vi "Step2.vi"(7 "Count In":i64, 8 "End":cluster{"Row":i32, "Col":i32}, 10 "Grid":string[][](array[string]), 11 "Current Pos":cluster{"Row":i32, "Col":i32}) -> (3 "Counts Out":i64[](array[numeric]))   [LabVIEW 2021]
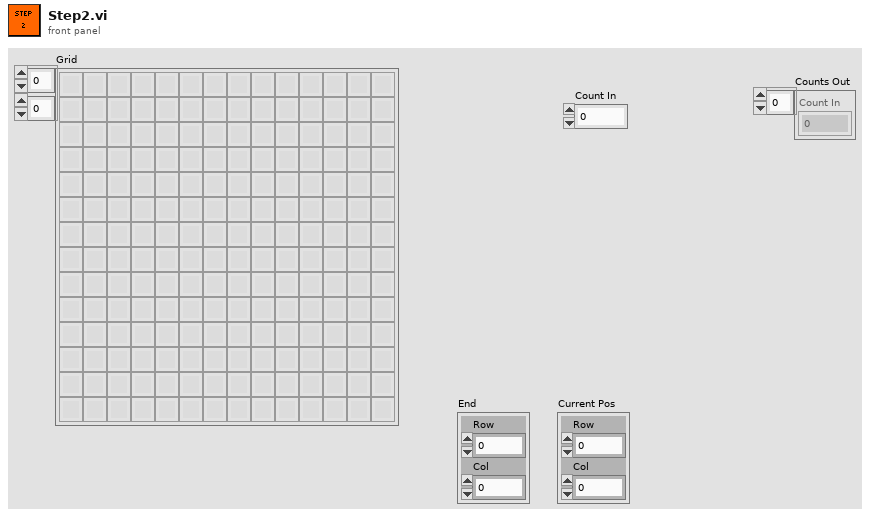
[diagram p1: front panel]
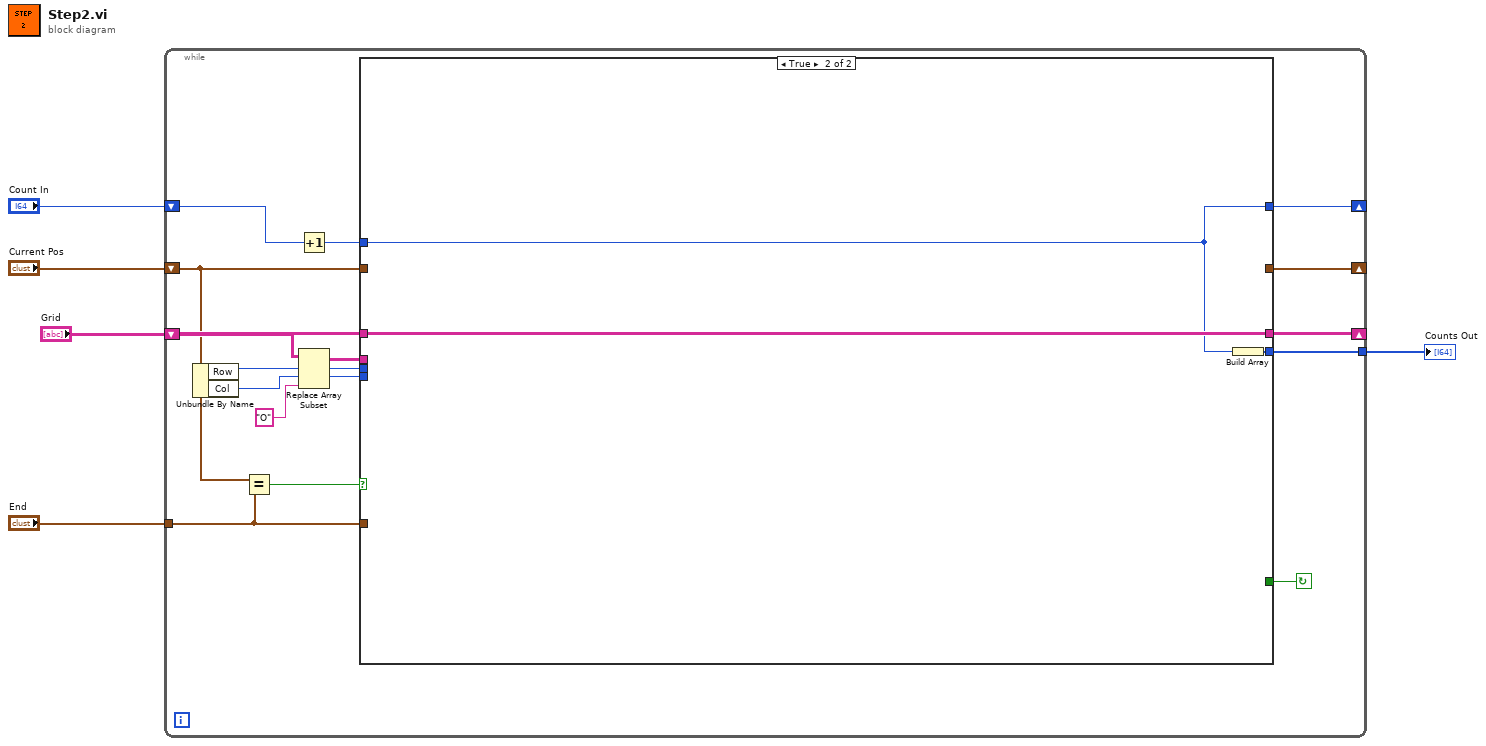
[diagram p0: block diagram]
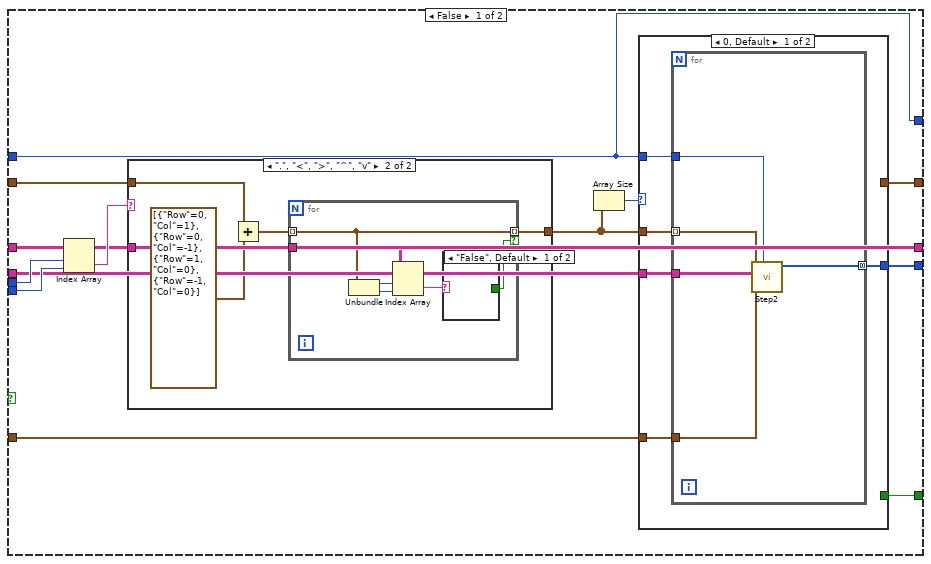
[diagram p2: hidden frame]
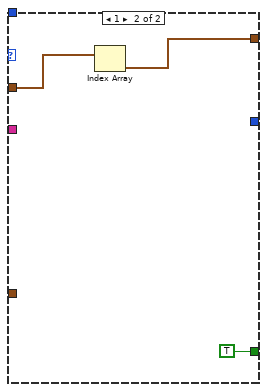
[diagram p3: hidden frame]
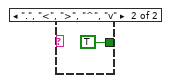
[diagram p5: hidden frame]
diagram:
  n1 = while {
    tunnel: [w20] -> w5
    tunnel: "End" -> [w16]
    shift-right: [w8] -> _
    shift-left: "Count In" -> [w12]
    shift-right: [w7] -> _
    shift-left: "Current Pos" -> [w10]
    shift-right: [w6] -> _
    shift-left: "Grid" -> [w13]
    stop <- w9 continue-if-true
    n2 = Unbundle By Name(w10) -> ("Row"=w15:i32, "Col"=w14:i32)
    n3 = Equal?(x=w10, y=w16) -> (x = y?=w17:bool)
    n4 = Increment(x=w12) -> (x+1=w11:i64)
    n5 = Replace Array Subset(array=w13, new element="O" ("new element/subarray"), index (row)=w15, index (col)=w14) -> (w18:string[][])
    n6 = case shown="False" w17 {
      tunnel: w11 -> [w23 w59]
      tunnel: [w33 w61] -> w20
      tunnel: w18 -> [w28 _]
      tunnel: w16 -> [w32 _]
      tunnel: w15 -> [w29 _]
      tunnel: w14 -> [w31 _]
      tunnel: w10 -> [w30 _]
      tunnel: w13 -> [w21 w60]
      tunnel: [w24 _] -> w9
      tunnel: [w23 w59] -> w8
      tunnel: [w22 _] -> w7
      tunnel: [w21 w60] -> w6
      frame False {
        n7 = Index Array(array=w21, index (row)=w29, index (col)=w31) -> (element=w27:string)
        n8 = case shown="\".\", \"<\", \">\", \"^\", \"v\"" w27 {
          tunnel: w30 -> [_ w51]
          tunnel: [_ w47] -> w26
          tunnel: w21 -> [_ w48]
          frame Default {
          }
          frame ".", "<", ">", "^", "v" {
            n9 = Add(x=w51, y=cluster{"Row":i32, "Col":i32}[] [{"Row"=0, "Col"=1}, {"Row"=0, "Col"=-1}, {"Row"=1, "Col"=0}, {"Row"=-1, "Col"=0}]) -> (x+y=w49:cluster{"Row":i32, "Col":i32}[])
            n10 = for {
              tunnel: w49 -> [w54] mode=indexing
              tunnel: w48 -> [w57]
              tunnel: [w54] -> w47 mode=indexing if=w52
              n11 = Unbundle(w54) -> ("Row"=w56:i32, "Col"=w55:i32)
              n12 = Index Array(array=w57, index (row)=w56, index (col)=w55) -> (element=w53:string)
              n13 = case shown="\"False\", Default" w53 {
                tunnel: [_ TRUE] -> w52
                frame "False", Default {
                }
                frame ".", "<", ">", "^", "v" {
                }
              }
            }
          }
        }
        n14 = Array Size(array=w26) -> (size(s)=w25:i32)
        n15 = case shown="0, Default" w25 {
          tunnel: w23 -> [w38 _]
          tunnel: [w37 _] -> w33
          tunnel: w32 -> [w36 _]
          tunnel: w28 -> [w35 _]
          tunnel: w26 -> [w34 w45]
          tunnel: [_ TRUE] -> w24
          tunnel: [_ w44] -> w22
          frame 0, Default {
            n16 = for {
              tunnel: w38 -> [w41]
              tunnel: [w43] -> w37 mode=concatenating
              tunnel: w35 -> [w42]
              tunnel: w36 -> [w40]
              tunnel: w34 -> [w39] mode=indexing
              n17 = call "Step2.vi"("Count In"=w41, "End"=w40, "Grid"=w42, "Current Pos"=w39) -> ("Counts Out"=w43:i64[])  [unwired: 7 in]
            }
          }
          frame 1 {
            n18 = Index Array(array=w45) -> (element=w44:cluster{"Row":i32, "Col":i32})  [unwired: 1 in]
          }
        }
      }
      frame True {
        n19 = Build Array(w59) -> (w61:i64[])
      }
    }
  }
  "Counts Out" <- w5
